vi "Calibration Key string to Calibration params Array.vi"(10 "Calibration Type":string, 11 "Key String IN":string) -> (1 "Imaging (Galvo/Reso) Key Array":T1[](array[typedef]), 2 "Photostim Galvo Key Array":T1[](array[typedef]), 3 "Image Pixels OUT":cluster{"X Pixels":i32, "Y Pixels":i32})   [LabVIEW 2012]
uses:
  Custom Controls and Typedefs/Calibration Key Param structure.ctl
  <vilib>/Utility/VariantDataType/Type.ctl
  Custom Controls and Typedefs/Galvo Key Parameters.ctl
  Custom Controls and Typedefs/Reso Key Parameters.ctl
  Custom Controls and Typedefs/Galvo (Stim Path) Key Parameters.ctl
  <vilib>/Utility/VariantDataType/VariantType.lvlib
panel:
  out "I Path Text Array":cluster{"GFG varname":string, "value":string}[](array[cluster])
  out "S Path Text Array":cluster{"GFG varname":string, "value":string}[](array[cluster])
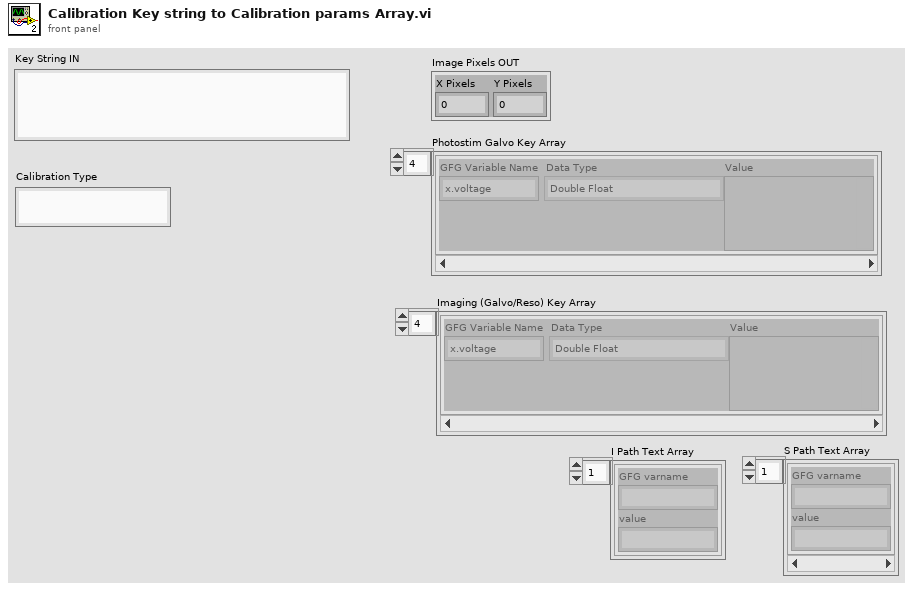
[diagram p1: front panel]
types:
  T1 = typedef "Calibration Key Param structure.ctl" = cluster{"GFG Variable Name":string, "Data Type":T2, "Value":variant}
  T2 = typedef "VariantType.lvlib/Type.ctl" = enum8{"Invalid Type", "Void", "I8", "I16", "I32", "I64", "U8", "U16", "U32", "U64", "Single Float", "Double Float", "Extended Float", "Single Complex", "Double Complex", "Extended Complex", "Enum U8", "Enum U16", "Enum U32", "Enum U64", "Single Float With Unit", "Double Float With Unit", "Extended Float With Unit", "Single Complex with Unit", "Double Complex with Unit", "Extended Complex with Unit", "Boolean", "String", "Path", "Picture", "Tag", "Array", "Cluster", "Variant", "LV Variant", "Waveform", "Timestamp", "Digital Waveform", "Digital Data", "ExpressData", "Refnum", "External Data", "VI", "Poly VI", "LabVIEW Class Instance", "Fixed Point"}
  T3 = typedef "Galvo (Stim Path) Key Parameters.ctl" = T1[]
  T4 = typedef "Reso Key Parameters.ctl" = T1[]
  T5 = typedef "Galvo Key Parameters.ctl" = T1[]
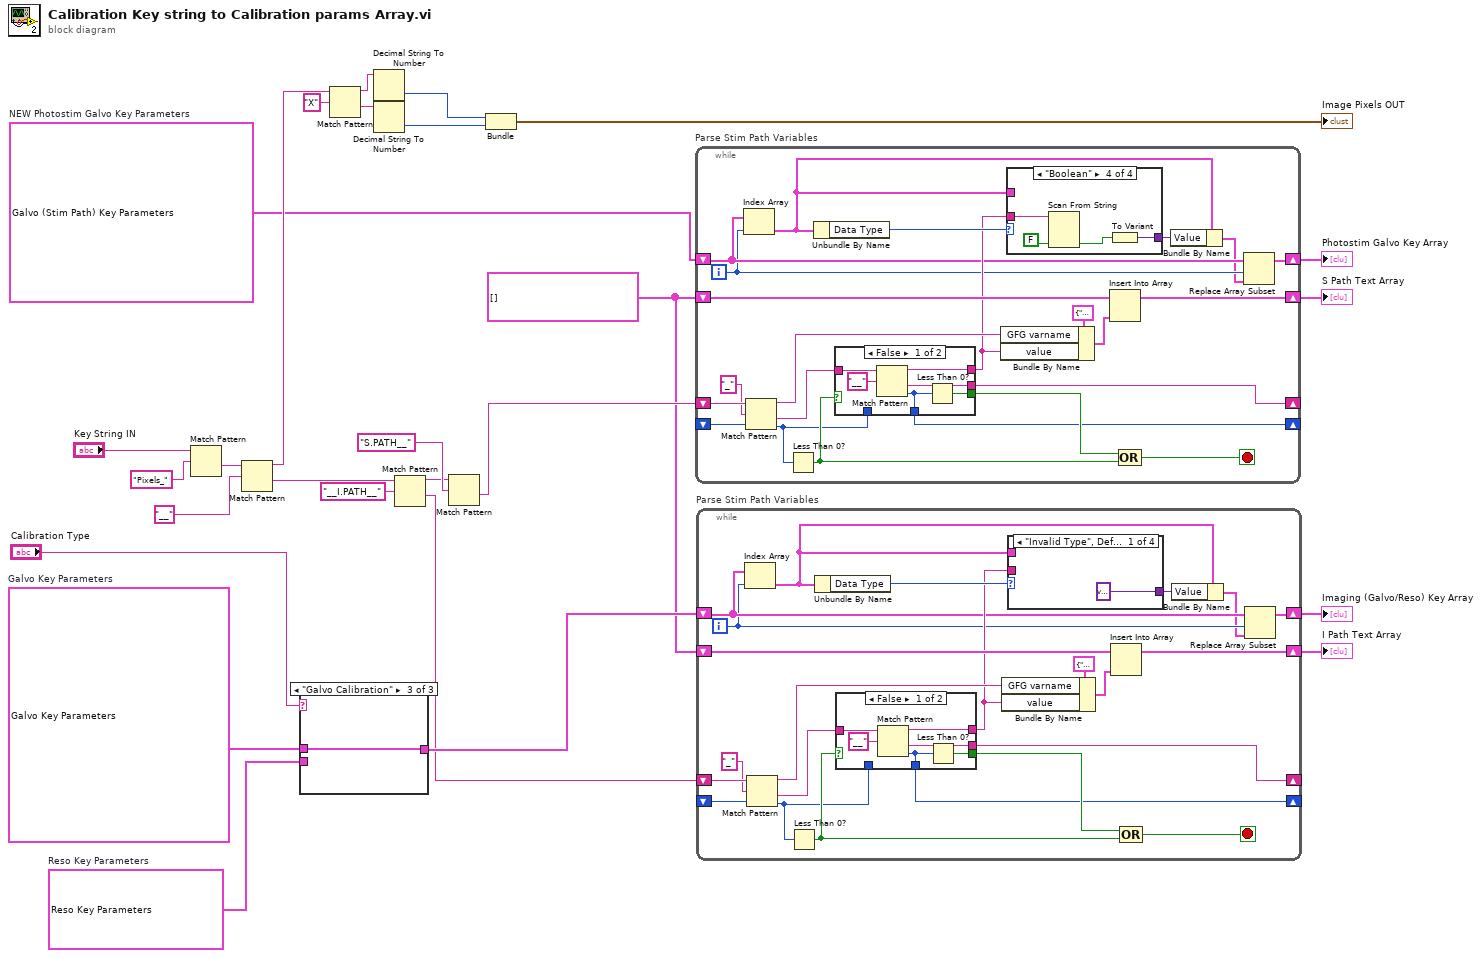
[diagram p0: block diagram]
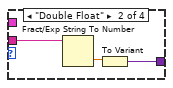
[diagram p2: hidden frame]
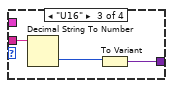
[diagram p3: hidden frame]
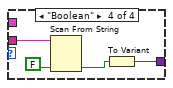
[diagram p4: hidden frame]
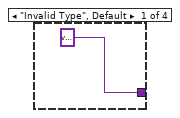
[diagram p8: hidden frame]
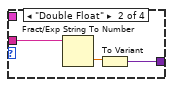
[diagram p9: hidden frame]
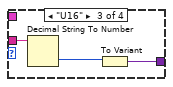
[diagram p10: hidden frame]
diagram:
  w1 = T3 [{"GFG Variable Name"="x.voltage", "Data Type"=enum."Double Float", "Value"=variant}, {"GFG Variable Name"="y.voltage", "Data Type"=enum."Double Float", "Value"=variant}, {"GFG Variable Name"="x.volt.offset", "Data Type"=enum."Double Float", "Value"=variant}, {"GFG Variable Name"="y.volt.offset", "Data Type"=enum."Double Float", "Value"=variant}, {"GFG Variable Name"="fill.fraction", "Data Type"=enum."Double Float", "Value"=variant}, {"GFG Variable Name"="x.invert.image", "Data Type"=enum."Boolean", "Value"=variant}, {"GFG Variable Name"="y.invert.image", "Data Type"=enum."Boolean", "Value"=variant}]  # NEW Photostim Galvo Key Parameters
  w11 = T4 [{"GFG Variable Name"="x.voltage", "Data Type"=enum."Double Float", "Value"=variant}, {"GFG Variable Name"="y.voltage", "Data Type"=enum."Double Float", "Value"=variant}, {"GFG Variable Name"="x.correction", "Data Type"=enum."Double Float", "Value"=variant}]  # Reso Key Parameters
  w12 = T5 [{"GFG Variable Name"="x.voltage", "Data Type"=enum."Double Float", "Value"=variant}, {"GFG Variable Name"="y.voltage", "Data Type"=enum."Double Float", "Value"=variant}, {"GFG Variable Name"="x.volt.offset", "Data Type"=enum."Double Float", "Value"=variant}, {"GFG Variable Name"="y.volt.offset", "Data Type"=enum."Double Float", "Value"=variant}, {"GFG Variable Name"="speed.mode", "Data Type"=enum."U16", "Value"=variant}, {"GFG Variable Name"="fill.fraction", "Data Type"=enum."Double Float", "Value"=variant}, {"GFG Variable Name"="x.bidirectional", "Data Type"=enum."Boolean", "Value"=variant}, {"GFG Variable Name"="y.bidirectional", "Data Type"=enum."Boolean", "Value"=variant}, {"GFG Variable Name"="x.invert.image", "Data Type"=enum."Boolean", "Value"=variant}, {"GFG Variable Name"="y.invert.image", "Data Type"=enum."Boolean", "Value"=variant}]  # Galvo Key Parameters
  w7 = cluster{"GFG varname":string, "value":string}[] []
  n1 = Match Pattern(string="Key String IN", regular expression="Pixels_") -> (after substring=w25:string)  [unwired: 1 in, 3 out]
  n2 = Match Pattern(string=w25, regular expression="__") -> (before substring=w23:string, after substring=w19:string)  [unwired: 1 in, 2 out]
  n3 = case shown="\"Galvo Calibration\"" "Calibration Type" {
    tunnel: w12 -> [_ _ w29]
    tunnel: w11 -> [_ w28 _]
    tunnel: [_ w28 w29] -> w9
    frame "False", Default {
    }
    frame "Reso Calibration" {
    }
    frame "Galvo Calibration" {
    }
  }
  n4 = Match Pattern(string=w23, regular expression="X") -> (before substring=w21:string, after substring=w20:string)  [unwired: 1 in, 2 out]
  n5 = Decimal String To Number(string=w21) -> (number=w4:i32)  [unwired: 2 in, 1 out]
  n6 = Decimal String To Number(string=w20) -> (number=w3:i32)  [unwired: 2 in, 1 out]
  n7 = Match Pattern(string=w19, regular expression="__I.PATH__") -> (before substring=w16:string, after substring=w8:string)  [unwired: 1 in, 2 out]
  n8 = Match Pattern(string=w16, regular expression="S.PATH__") -> (after substring=w14:string)  [unwired: 1 in, 3 out]
  n9 = Bundle(w4, w3) -> (→"Image Pixels OUT":cluster{i32, i32})  [unwired: 1 in]
  n10 = while "Parse Stim Path Variables" {
    shift-right: [w40] -> _
    shift-left: _ -> [w49]
    shift-right: [w44] -> w15
    shift-left: w7 -> [w46]
    shift-right: [w41] -> _
    shift-left: w14 -> [w51]
    shift-right: [w30] -> w10
    shift-left: w1 -> [w33]
    i -> [w32]
    stop <- w52 stop-if-true
    n11 = Index Array(array=w33, index=w32) -> (element=w34:T1)
    n12 = Match Pattern(string=w51, regular expression="_", offset (0)=w49) -> (before substring=w43:string, after substring=w42:string, offset past match=w39:i32)  [unwired: 1 out]
    n13 = Less Than 0?(x=w39) -> (x < 0?=w48:bool)
    n14 = Unbundle By Name(w34) -> ("Data Type"=w37:T2)
    n15 = case shown="False" w48 {
      tunnel: w42 -> [w69 w71]
      tunnel: [w67 _] -> w47
      tunnel: [w66 w71] -> w36
      tunnel: [w65 w71] -> w41
      tunnel: [w64 w70] -> w40
      tunnel: w39 -> [_ w70]
      frame False {
        n16 = Match Pattern(string=w69, regular expression="__") -> (before substring=w66:string, after substring=w65:string, offset past match=w64:i32)  [unwired: 1 in, 1 out]
        n17 = Less Than 0?(x=w64) -> (x < 0?=w67:bool)
      }
      frame True {
      }
    }
    n18 = Bundle By Name(cluster=cluster{"GFG varname":string, "value":string} {"GFG varname"="", "value"=""}, "GFG varname"=w43, "value"=w36) -> (w45:cluster{"GFG varname":string, "value":string})
    n19 = case shown="\"Boolean\"" w37 {
      tunnel: w36 -> [_ w56 w58 w63]
      tunnel: w34 -> [_ _ _ _]
      tunnel: [variant ("Value") w54 w59 w60] -> w35
      frame "Invalid Type", Default {
      }
      frame "Double Float" {
        n20 = Fract/Exp String To Number(string=w56) -> (number=w55:dbl)  [unwired: 3 in, 1 out]
        n21 = To Variant(anything=w55) -> (Variant=w54:variant)
      }
      frame "U16" {
        n22 = Decimal String To Number(string=w58) -> (number=w57:i32)  [unwired: 2 in, 1 out]
        n23 = To Variant(anything=w57) -> (Variant=w59:variant)
      }
      frame "Boolean" {
        n24 = Scan From String(input string=w63, default 1=FALSE) -> (output 1=w61:bool)  [unwired: 3 in, 3 out]
        n25 = To Variant(anything=w61) -> (Variant=w60:variant)
      }
    }
    n26 = Insert Into Array(array=w46, new element=w45) -> (w44:cluster{"GFG varname":string, "value":string}[])  [unwired: 1 in]
    n27 = Compound Arithmetic op=OR(w47, w48) -> (w52:bool)
    n28 = Bundle By Name(cluster=w34, "Value"=w35) -> (w31:T1)
    n29 = Replace Array Subset(array=w33, new element=w31, index=w32) -> (w30:T3)
  }
  "S Path Text Array" <- w15
  "Photostim Galvo Key Array" <- w10
  n30 = while "Parse Stim Path Variables" {
    shift-right: [w82] -> _
    shift-left: _ -> [w91]
    shift-right: [w86] -> w5
    shift-left: w7 -> [w88]
    shift-right: [w83] -> _
    shift-left: w8 -> [w93]
    shift-right: [w72] -> w6
    shift-left: w9 -> [w75]
    i -> [w74]
    stop <- w94 stop-if-true
    n31 = Index Array(array=w75, index=w74) -> (element=w76:T1)
    n32 = Match Pattern(string=w93, regular expression="_", offset (0)=w91) -> (before substring=w85:string, after substring=w84:string, offset past match=w81:i32)  [unwired: 1 out]
    n33 = Less Than 0?(x=w81) -> (x < 0?=w90:bool)
    n34 = Unbundle By Name(w76) -> ("Data Type"=w79:T2)
    n35 = case shown="False" w90 {
      tunnel: w84 -> [w111 w113]
      tunnel: [w109 _] -> w89
      tunnel: [w108 w113] -> w78
      tunnel: [w107 w113] -> w83
      tunnel: [w106 w112] -> w82
      tunnel: w81 -> [_ w112]
      frame False {
        n36 = Match Pattern(string=w111, regular expression="__") -> (before substring=w108:string, after substring=w107:string, offset past match=w106:i32)  [unwired: 1 in, 1 out]
        n37 = Less Than 0?(x=w106) -> (x < 0?=w109:bool)
      }
      frame True {
      }
    }
    n38 = Bundle By Name(cluster=cluster{"GFG varname":string, "value":string} {"GFG varname"="", "value"=""}, "GFG varname"=w85, "value"=w78) -> (w87:cluster{"GFG varname":string, "value":string})
    n39 = case shown="\"Invalid Type\", Default" w79 {
      tunnel: w78 -> [_ w98 w100 w105]
      tunnel: w76 -> [_ _ _ _]
      tunnel: [variant ("Value") w96 w101 w102] -> w77
      frame "Invalid Type", Default {
      }
      frame "Double Float" {
        n40 = Fract/Exp String To Number(string=w98) -> (number=w97:dbl)  [unwired: 3 in, 1 out]
        n41 = To Variant(anything=w97) -> (Variant=w96:variant)
      }
      frame "U16" {
        n42 = Decimal String To Number(string=w100) -> (number=w99:i32)  [unwired: 2 in, 1 out]
        n43 = To Variant(anything=w99) -> (Variant=w101:variant)
      }
      frame "Boolean" {
        n44 = Scan From String(input string=w105, default 1=FALSE) -> (output 1=w103:bool)  [unwired: 3 in, 3 out]
        n45 = To Variant(anything=w103) -> (Variant=w102:variant)
      }
    }
    n46 = Insert Into Array(array=w88, new element=w87) -> (w86:cluster{"GFG varname":string, "value":string}[])  [unwired: 1 in]
    n47 = Compound Arithmetic op=OR(w89, w90) -> (w94:bool)
    n48 = Bundle By Name(cluster=w76, "Value"=w77) -> (w73:T1)
    n49 = Replace Array Subset(array=w75, new element=w73, index=w74) -> (w72:T5)
  }
  "Imaging (Galvo/Reso) Key Array" <- w6
  "I Path Text Array" <- w5
